vi "TestExec.Set Station Notification.vi"(7 "Module Q Name":string, 8 "error in":errorcluster, 10 "Notification En":bool, 11 "Q In":refnum<queue>) -> (0 "error out":errorcluster)   [LabVIEW 2018]
uses:
  <vilib>/KATE/Queues/Q.Element.ctl
  <vilib>/KATE/Queues/Queue Utils.lvlib
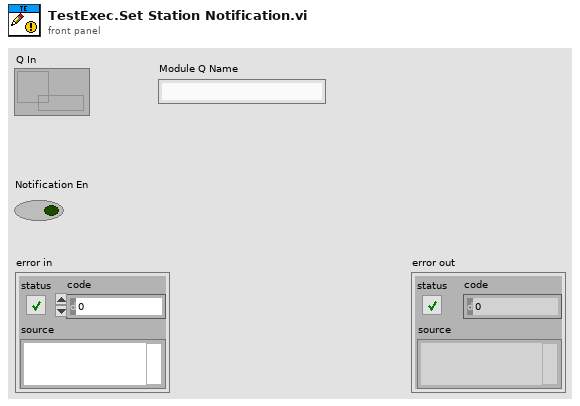
[diagram p1: front panel]
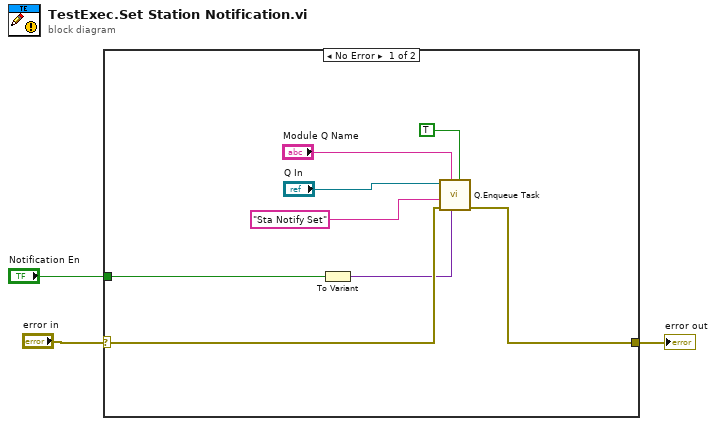
[diagram p0: block diagram]
diagram:
  n1 = case shown="No Error" "error in" {
    selector: "error in" -> [w8 w12]
    tunnel: [w9 w12] -> w2
    tunnel: "Notification En" -> [w4 _]
    frame No Error {
      n2 = To Variant(anything=w4) -> (Variant=w7:variant)
      n3 = call <vilib>:"Q.Enqueue Task.vi"("Top of Q"=TRUE, "Data1"=w7, "Q Name"="Module Q Name", "Error In"=w8, "Task Name"="Sta Notify Set" ("Cmd"), "Q In"="Q In") -> ("error out"=w9:errorcluster)  [unwired: 4 in, 1 out]
    }
    frame Error {
    }
  }
  "error out" <- w2
